vi "InitGoalFields.vi"(9 "3rdShiftConfig":T1={"StartHour"=[{"Hour"=5, "Minute"=0}, {"Hour"=6, "Minute"=0}, {"Hour"=7, "Minute"=0}, {"Hour"=7, "Minute"=30}, {"Hour"=0, "Minute"=0}, {"Hour"=0, "Minute"=0}, {"Hour"=0, "Minute"=0}, {"Hour"=0, "Minute"=0}, {"Hour"=0, "Minute"=0}], "Goal"=[], "EndHour"=[{"Hour"=5, "Minute"=59}, {"Hour"=6, "Minute"=59}, {"Hour"=7, "Minute"=10}, {"Hour"=7, "Minute"=59}, {"Hour"=0, "Minute"=0}, {"Hour"=0, "Minute"=0}, {"Hour"=0, "Minute"=0}, {"Hour"=0, "Minute"=0}, {"Hour"=0, "Minute"=0}], "AM/PM"=[]} caption="3rdShift" {"AM/PM"."AM/PM" items=["AM", "PM"]; "EndHour"."Minute" items=["00", "1", "2", "3", "4", "5", "6", "7", "8", "9", "10", "11", "12", "13", "14", "15", "16", "17", "18", "19", "20", "21", "22", "23", "24", "25", "26", "27", "28", "29", "30", "31", "32", "33", "34", "35", "36", "37", "38", "39", "40", "41", "42", "43", "44", "45", "46", "47", "48", "49", "50", "51", "52", "53", "54", "55", "56", "57", "58", "59"]; "EndHour"."Hour" items=["0", "1", "2", "3", "4", "5", "6", "7", "8", "9", "10", "11", "12", "13", "14", "15", "16", "17", "18", "19", "20", "21", "22", "23"]; "StartHour"."Minute" items=["00", "1", "2", "3", "4", "5", "6", "7", "8", "9", "10", "11", "12", "13", "14", "15", "16", "17", "18", "19", "20", "21", "22", "23", "24", "25", "26", "27", "28", "29", "30", "31", "32", "33", "34", "35", "36", "37", "38", "39", "40", "41", "42", "43", "44", "45", "46", "47", "48", "49", "50", "51", "52", "53", "54", "55", "56", "57", "58", "59"]; "StartHour"."Hour" items=["0", "1", "2", "3", "4", "5", "6", "7", "8", "9", "10", "11", "12", "13", "14", "15", "16", "17", "18", "19", "20", "21", "22", "23"]}, 10 "2ndShiftConfig":T1={"StartHour"=[{"Hour"=5, "Minute"=0}, {"Hour"=6, "Minute"=0}, {"Hour"=7, "Minute"=0}, {"Hour"=7, "Minute"=30}, {"Hour"=0, "Minute"=0}, {"Hour"=0, "Minute"=0}, {"Hour"=0, "Minute"=0}, {"Hour"=0, "Minute"=0}, {"Hour"=0, "Minute"=0}], "Goal"=[], "EndHour"=[{"Hour"=5, "Minute"=59}, {"Hour"=6, "Minute"=59}, {"Hour"=7, "Minute"=10}, {"Hour"=7, "Minute"=59}, {"Hour"=0, "Minute"=0}, {"Hour"=0, "Minute"=0}, {"Hour"=0, "Minute"=0}, {"Hour"=0, "Minute"=0}, {"Hour"=0, "Minute"=0}], "AM/PM"=[{"AM/PM"=1}, {"AM/PM"=1}, {"AM/PM"=1}, {"AM/PM"=1}, {"AM/PM"=1}, {"AM/PM"=1}, {"AM/PM"=1}, {"AM/PM"=1}, {"AM/PM"=1}]} caption="2ndShift" {"AM/PM"."AM/PM" items=["AM", "PM"]; "EndHour"."Minute" items=["00", "1", "2", "3", "4", "5", "6", "7", "8", "9", "10", "11", "12", "13", "14", "15", "16", "17", "18", "19", "20", "21", "22", "23", "24", "25", "26", "27", "28", "29", "30", "31", "32", "33", "34", "35", "36", "37", "38", "39", "40", "41", "42", "43", "44", "45", "46", "47", "48", "49", "50", "51", "52", "53", "54", "55", "56", "57", "58", "59"]; "EndHour"."Hour" items=["00", "1", "2", "3", "4", "5", "6", "7", "8", "9", "10", "11", "12", "13", "14", "15", "16", "17", "18", "19", "20", "21", "22", "23"]; "StartHour"."Minute" items=["00", "1", "2", "3", "4", "5", "6", "7", "8", "9", "10", "11", "12", "13", "14", "15", "16", "17", "18", "19", "20", "21", "22", "23", "24", "25", "26", "27", "28", "29", "30", "31", "32", "33", "34", "35", "36", "37", "38", "39", "40", "41", "42", "43", "44", "45", "46", "47", "48", "49", "50", "51", "52", "53", "54", "55", "56", "57", "58", "59"]; "StartHour"."Hour" items=["0", "1", "2", "3", "4", "5", "6", "7", "8", "9", "10", "11", "12", "13", "14", "15", "16", "17", "18", "19", "20", "21", "22", "23"]}, 11 "1stShiftConfig":T1={"StartHour"=[{"Hour"=5, "Minute"=0}, {"Hour"=6, "Minute"=0}, {"Hour"=7, "Minute"=0}, {"Hour"=7, "Minute"=30}, {"Hour"=0, "Minute"=0}, {"Hour"=0, "Minute"=0}, {"Hour"=0, "Minute"=0}, {"Hour"=0, "Minute"=0}, {"Hour"=0, "Minute"=0}], "Goal"=[], "EndHour"=[{"Hour"=5, "Minute"=59}, {"Hour"=6, "Minute"=59}, {"Hour"=7, "Minute"=10}, {"Hour"=7, "Minute"=59}, {"Hour"=0, "Minute"=0}, {"Hour"=0, "Minute"=0}, {"Hour"=0, "Minute"=0}, {"Hour"=0, "Minute"=0}, {"Hour"=0, "Minute"=0}], "AM/PM"=[{"AM/PM"=0}, {"AM/PM"=0}, {"AM/PM"=0}, {"AM/PM"=0}, {"AM/PM"=0}, {"AM/PM"=0}, {"AM/PM"=0}, {"AM/PM"=0}, {"AM/PM"=0}]} caption="1stShift" {"AM/PM"."AM/PM" items=["AM", "PM"]; "EndHour"."Minute" items=["00", "1", "2", "3", "4", "5", "6", "7", "8", "9", "10", "11", "12", "13", "14", "15", "16", "17", "18", "19", "20", "21", "22", "23", "24", "25", "26", "27", "28", "29", "30", "31", "32", "33", "34", "35", "36", "37", "38", "39", "40", "41", "42", "43", "44", "45", "46", "47", "48", "49", "50", "51", "52", "53", "54", "55", "56", "57", "58", "59"]; "EndHour"."Hour" items=["0", "1", "2", "3", "4", "5", "6", "7", "8", "9", "10", "11", "12", "13", "14", "15", "16", "17", "18", "19", "20", "21", "22", "23"]; "StartHour"."Minute" items=["00", "1", "2", "3", "4", "5", "6", "7", "8", "9", "10", "11", "12", "13", "14", "15", "16", "17", "18", "19", "20", "21", "22", "23", "24", "25", "26", "27", "28", "29", "30", "31", "32", "33", "34", "35", "36", "37", "38", "39", "40", "41", "42", "43", "44", "45", "46", "47", "48", "49", "50", "51", "52", "53", "54", "55", "56", "57", "58", "59"]; "StartHour"."Hour" items=["0", "1", "2", "3", "4", "5", "6", "7", "8", "9", "10", "11", "12", "13", "14", "15", "16", "17", "18", "19", "20", "21", "22", "23"]}) -> (1 "3rdShiftConfig 2":T1={"StartHour"=[{"Hour"=5, "Minute"=0}, {"Hour"=6, "Minute"=0}, {"Hour"=7, "Minute"=0}, {"Hour"=7, "Minute"=30}, {"Hour"=0, "Minute"=0}, {"Hour"=0, "Minute"=0}, {"Hour"=0, "Minute"=0}, {"Hour"=0, "Minute"=0}, {"Hour"=0, "Minute"=0}], "Goal"=[], "EndHour"=[{"Hour"=5, "Minute"=59}, {"Hour"=6, "Minute"=59}, {"Hour"=7, "Minute"=10}, {"Hour"=7, "Minute"=59}, {"Hour"=0, "Minute"=0}, {"Hour"=0, "Minute"=0}, {"Hour"=0, "Minute"=0}, {"Hour"=0, "Minute"=0}, {"Hour"=0, "Minute"=0}], "AM/PM"=[]} caption="3rdShift" {"AM/PM"."AM/PM" items=["AM", "PM"]; "EndHour"."Minute" items=["00", "1", "2", "3", "4", "5", "6", "7", "8", "9", "10", "11", "12", "13", "14", "15", "16", "17", "18", "19", "20", "21", "22", "23", "24", "25", "26", "27", "28", "29", "30", "31", "32", "33", "34", "35", "36", "37", "38", "39", "40", "41", "42", "43", "44", "45", "46", "47", "48", "49", "50", "51", "52", "53", "54", "55", "56", "57", "58", "59"]; "EndHour"."Hour" items=["0", "1", "2", "3", "4", "5", "6", "7", "8", "9", "10", "11", "12", "13", "14", "15", "16", "17", "18", "19", "20", "21", "22", "23"]; "StartHour"."Minute" items=["00", "1", "2", "3", "4", "5", "6", "7", "8", "9", "10", "11", "12", "13", "14", "15", "16", "17", "18", "19", "20", "21", "22", "23", "24", "25", "26", "27", "28", "29", "30", "31", "32", "33", "34", "35", "36", "37", "38", "39", "40", "41", "42", "43", "44", "45", "46", "47", "48", "49", "50", "51", "52", "53", "54", "55", "56", "57", "58", "59"]; "StartHour"."Hour" items=["0", "1", "2", "3", "4", "5", "6", "7", "8", "9", "10", "11", "12", "13", "14", "15", "16", "17", "18", "19", "20", "21", "22", "23"]}, 2 "2ndShiftConfig 2":T1={"StartHour"=[{"Hour"=5, "Minute"=0}, {"Hour"=6, "Minute"=0}, {"Hour"=7, "Minute"=0}, {"Hour"=7, "Minute"=30}, {"Hour"=0, "Minute"=0}, {"Hour"=0, "Minute"=0}, {"Hour"=0, "Minute"=0}, {"Hour"=0, "Minute"=0}, {"Hour"=0, "Minute"=0}], "Goal"=[], "EndHour"=[{"Hour"=5, "Minute"=59}, {"Hour"=6, "Minute"=59}, {"Hour"=7, "Minute"=10}, {"Hour"=7, "Minute"=59}, {"Hour"=0, "Minute"=0}, {"Hour"=0, "Minute"=0}, {"Hour"=0, "Minute"=0}, {"Hour"=0, "Minute"=0}, {"Hour"=0, "Minute"=0}], "AM/PM"=[{"AM/PM"=1}, {"AM/PM"=1}, {"AM/PM"=1}, {"AM/PM"=1}, {"AM/PM"=1}, {"AM/PM"=1}, {"AM/PM"=1}, {"AM/PM"=1}, {"AM/PM"=1}]} caption="2ndShift" {"AM/PM"."AM/PM" items=["AM", "PM"]; "EndHour"."Minute" items=["00", "1", "2", "3", "4", "5", "6", "7", "8", "9", "10", "11", "12", "13", "14", "15", "16", "17", "18", "19", "20", "21", "22", "23", "24", "25", "26", "27", "28", "29", "30", "31", "32", "33", "34", "35", "36", "37", "38", "39", "40", "41", "42", "43", "44", "45", "46", "47", "48", "49", "50", "51", "52", "53", "54", "55", "56", "57", "58", "59"]; "EndHour"."Hour" items=["00", "1", "2", "3", "4", "5", "6", "7", "8", "9", "10", "11", "12", "13", "14", "15", "16", "17", "18", "19", "20", "21", "22", "23"]; "StartHour"."Minute" items=["00", "1", "2", "3", "4", "5", "6", "7", "8", "9", "10", "11", "12", "13", "14", "15", "16", "17", "18", "19", "20", "21", "22", "23", "24", "25", "26", "27", "28", "29", "30", "31", "32", "33", "34", "35", "36", "37", "38", "39", "40", "41", "42", "43", "44", "45", "46", "47", "48", "49", "50", "51", "52", "53", "54", "55", "56", "57", "58", "59"]; "StartHour"."Hour" items=["0", "1", "2", "3", "4", "5", "6", "7", "8", "9", "10", "11", "12", "13", "14", "15", "16", "17", "18", "19", "20", "21", "22", "23"]}, 3 "1stShiftConfig 2":T1={"StartHour"=[{"Hour"=5, "Minute"=0}, {"Hour"=6, "Minute"=0}, {"Hour"=7, "Minute"=0}, {"Hour"=7, "Minute"=30}, {"Hour"=0, "Minute"=0}, {"Hour"=0, "Minute"=0}, {"Hour"=0, "Minute"=0}, {"Hour"=0, "Minute"=0}, {"Hour"=0, "Minute"=0}], "Goal"=[], "EndHour"=[{"Hour"=5, "Minute"=59}, {"Hour"=6, "Minute"=59}, {"Hour"=7, "Minute"=10}, {"Hour"=7, "Minute"=59}, {"Hour"=0, "Minute"=0}, {"Hour"=0, "Minute"=0}, {"Hour"=0, "Minute"=0}, {"Hour"=0, "Minute"=0}, {"Hour"=0, "Minute"=0}], "AM/PM"=[{"AM/PM"=0}, {"AM/PM"=0}, {"AM/PM"=0}, {"AM/PM"=0}, {"AM/PM"=0}, {"AM/PM"=0}, {"AM/PM"=0}, {"AM/PM"=0}, {"AM/PM"=0}]} caption="1stShift" {"AM/PM"."AM/PM" items=["AM", "PM"]; "EndHour"."Minute" items=["00", "1", "2", "3", "4", "5", "6", "7", "8", "9", "10", "11", "12", "13", "14", "15", "16", "17", "18", "19", "20", "21", "22", "23", "24", "25", "26", "27", "28", "29", "30", "31", "32", "33", "34", "35", "36", "37", "38", "39", "40", "41", "42", "43", "44", "45", "46", "47", "48", "49", "50", "51", "52", "53", "54", "55", "56", "57", "58", "59"]; "EndHour"."Hour" items=["0", "1", "2", "3", "4", "5", "6", "7", "8", "9", "10", "11", "12", "13", "14", "15", "16", "17", "18", "19", "20", "21", "22", "23"]; "StartHour"."Minute" items=["00", "1", "2", "3", "4", "5", "6", "7", "8", "9", "10", "11", "12", "13", "14", "15", "16", "17", "18", "19", "20", "21", "22", "23", "24", "25", "26", "27", "28", "29", "30", "31", "32", "33", "34", "35", "36", "37", "38", "39", "40", "41", "42", "43", "44", "45", "46", "47", "48", "49", "50", "51", "52", "53", "54", "55", "56", "57", "58", "59"]; "StartHour"."Hour" items=["0", "1", "2", "3", "4", "5", "6", "7", "8", "9", "10", "11", "12", "13", "14", "15", "16", "17", "18", "19", "20", "21", "22", "23"]})   [LabVIEW 2017]
panel:
  in  "Cluster":cluster{"Goal":dbl}
  # "IN"
  # "OUT"
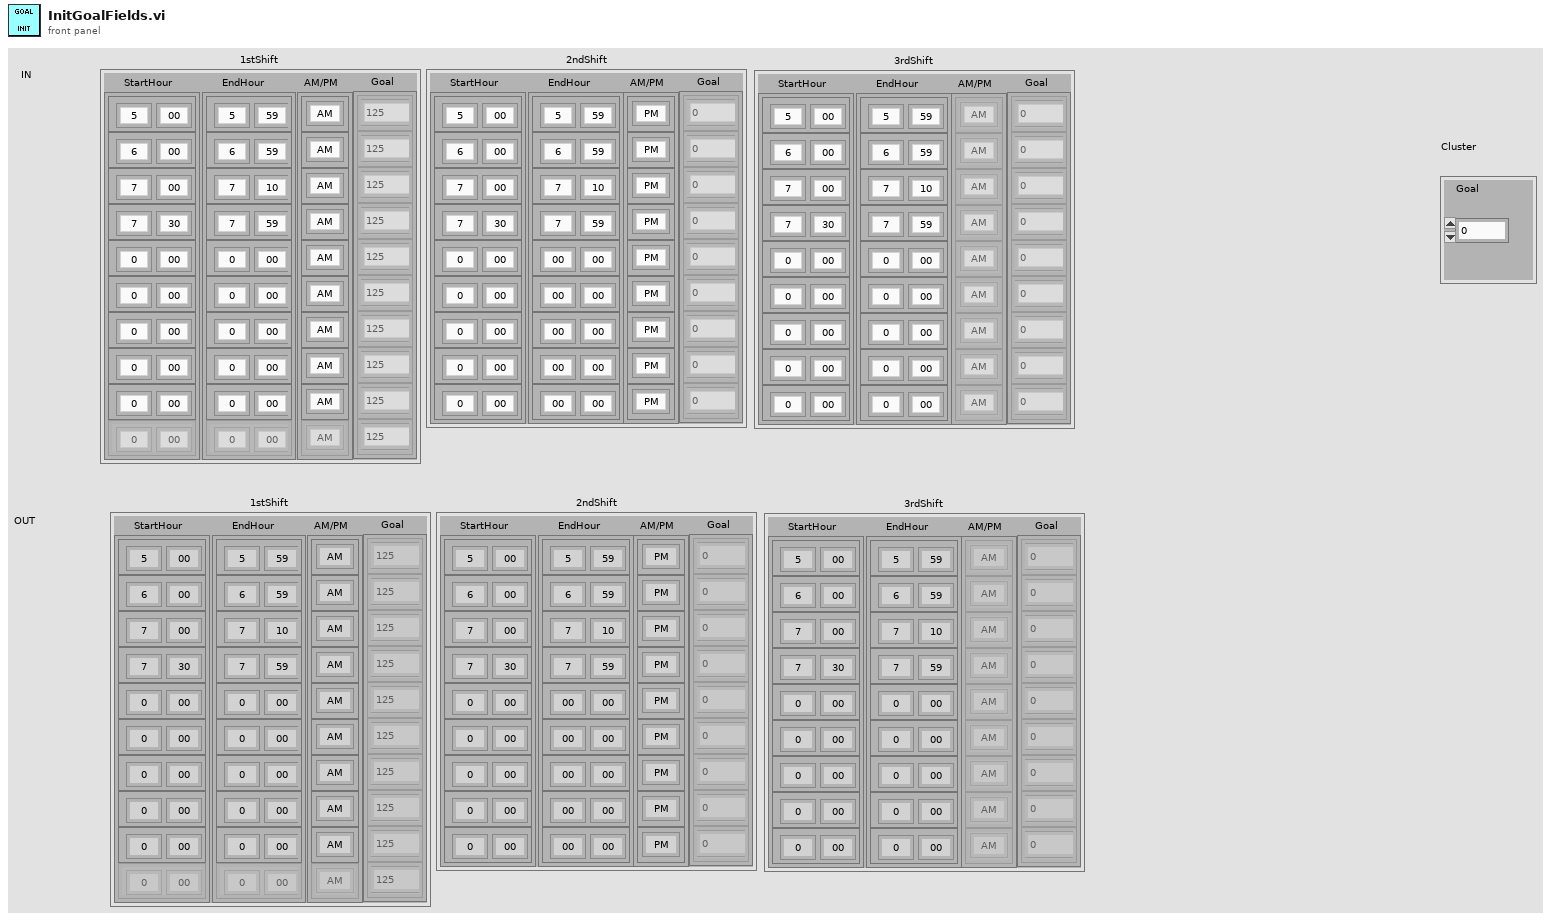
[diagram p1: front panel]
types:
  T1 = cluster{"StartHour":cluster{"Hour":u16, "Minute":u16}[], "Goal":cluster{"Goal":dbl}[], "EndHour":cluster{"Hour":u16, "Minute":u16}[], "AM/PM":cluster{"AM/PM":u16}[]}
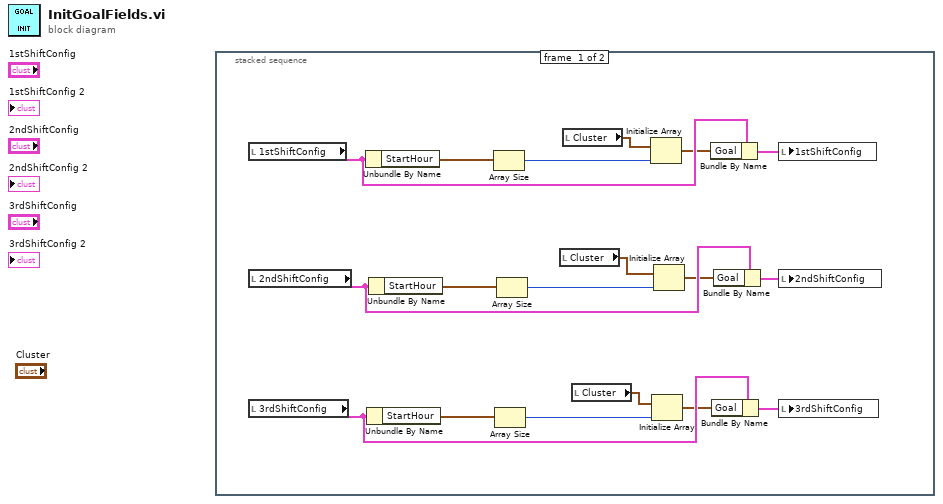
[diagram p0: block diagram]
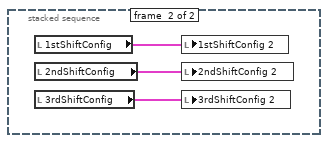
[diagram p2: hidden frame]
diagram:
  n1 = stacked-sequence {
    frame #0 {
      n2 = local read "1stShiftConfig"() -> (w16:T1)
      n3 = local read "2ndShiftConfig"() -> (w13:T1)
      n4 = local read "3rdShiftConfig"() -> (w8:T1)
      n5 = Unbundle By Name(w16) -> ("StartHour"=w17:cluster{"Hour":u16, "Minute":u16}[])
      n6 = Unbundle By Name(w8) -> ("StartHour"=w9:cluster{"Hour":u16, "Minute":u16}[])
      n7 = Unbundle By Name(w13) -> ("StartHour"=w12:cluster{"Hour":u16, "Minute":u16}[])
      n8 = Array Size(array=w17) -> (size(s)=w18:i32)
      n9 = Array Size(array=w9) -> (size(s)=w10:i32)
      n10 = Array Size(array=w12) -> (size(s)=w11:i32)
      n11 = local read "Cluster"() -> (w6:cluster{"Goal":dbl})
      n12 = local read "Cluster"() -> (w5:cluster{"Goal":dbl})
      n13 = local read "Cluster"() -> (w4:cluster{"Goal":dbl})
      n14 = Initialize Array(w5, w18) -> (w2:cluster{"Goal":dbl}[])
      n15 = Initialize Array(w4, w10) -> (w1:cluster{"Goal":dbl}[])
      n16 = Initialize Array(w6, w11) -> (w3:cluster{"Goal":dbl}[])
      n17 = Bundle By Name(cluster=w16, "Goal"=w2) -> (w15:T1)
      n18 = Bundle By Name(cluster=w8, "Goal"=w1) -> (w7:T1)
      n19 = Bundle By Name(cluster=w13, "Goal"=w3) -> (w14:T1)
      n20 = local write "1stShiftConfig"(w15) -> ()
      n21 = local write "2ndShiftConfig"(w14) -> ()
      n22 = local write "3rdShiftConfig"(w7) -> ()
    }
    frame #1 {
      n23 = local read "1stShiftConfig"() -> (w19:T1)
      n24 = local read "2ndShiftConfig"() -> (w20:T1)
      n25 = local read "3rdShiftConfig"() -> (w21:T1)
      n26 = local write "1stShiftConfig 2"(w19) -> ()
      n27 = local write "2ndShiftConfig 2"(w20) -> ()
      n28 = local write "3rdShiftConfig 2"(w21) -> ()
    }
  }
